vi "Output Powers.vi"(8 "error in":errorcluster, 9 "connection information":path, 10 "System Number":string, 11 "Arduino in":refnum<visa-resource-name>) -> (0 "error out":errorcluster, 3 "Arduino out":refnum<visa-resource-name>)   [LabVIEW 2024]
uses:
  <vilib>/addons/database/Connection.llb/DB Tools Open Connec (Path).vi
  <vilib>/addons/database/_DB Variant To Data/Database Variant To Data.xnode
  <instrlib>/Rohde&Schwarz Power Meter/Rohde&Schwarz Power Meter.lvlib
  <vilib>/addons/database/NI_Database_API.lvlib
panel:
  out "EFCVoltage":string
  out "OscVoltage":string
  out "Command Array":string[](array[string])
  out "OutputPower":string
  out "Temperature":string
  out "Nominal Frequency":string
  in  "DC_SN":string
  out "IsSine":bool=TRUE
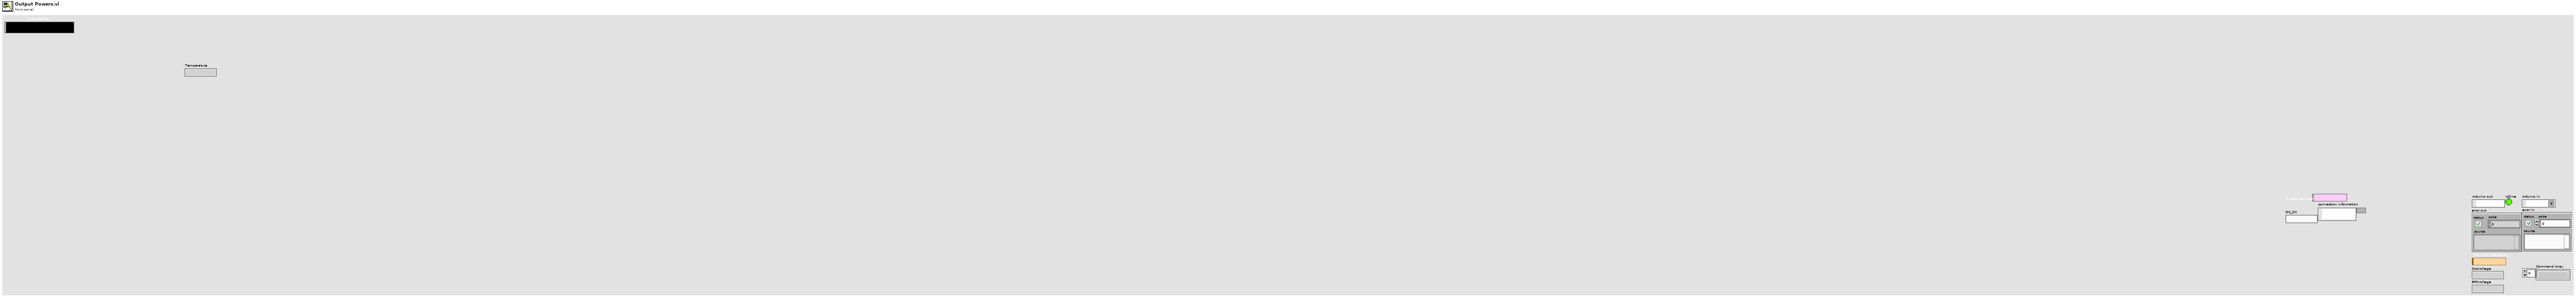
[diagram p1: front panel]
types:
  T1 = typedef "NI_Database_API.lvlib/Conn ObjectReference.ctl" = refnum<k1>
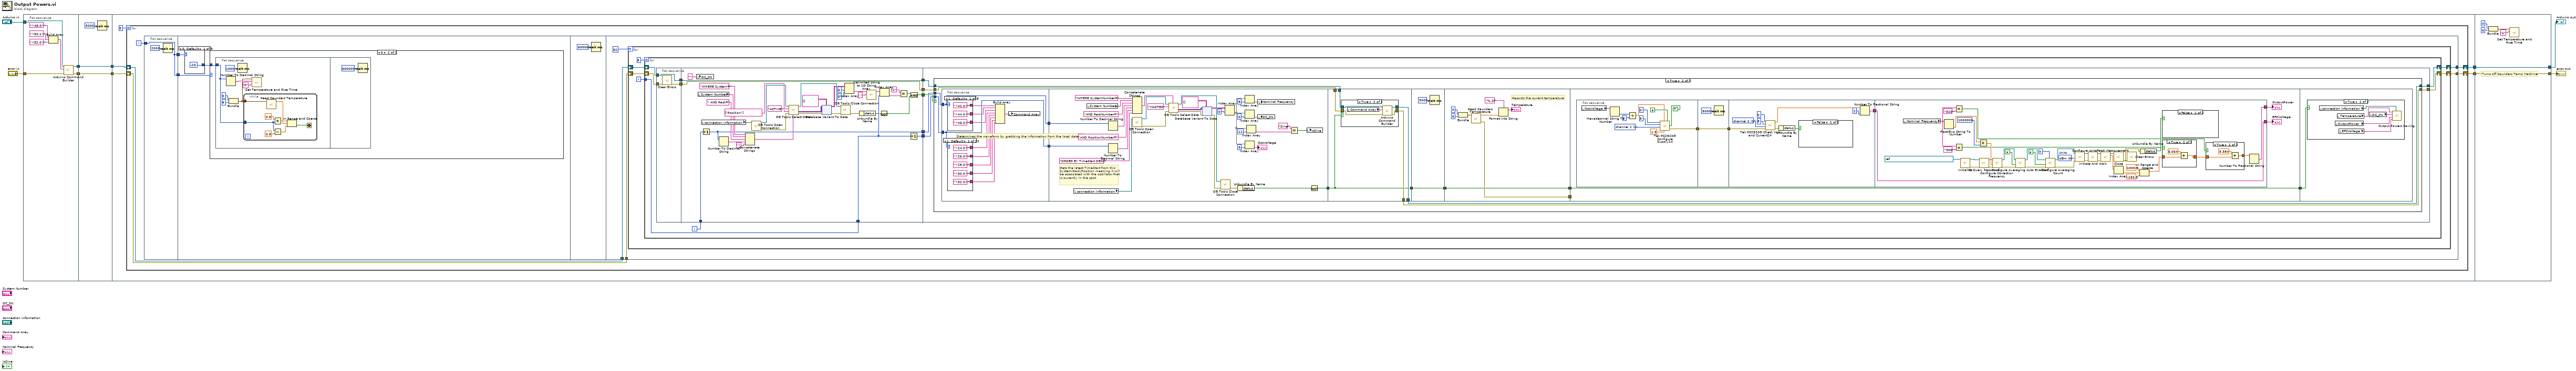
[diagram p0: block diagram]
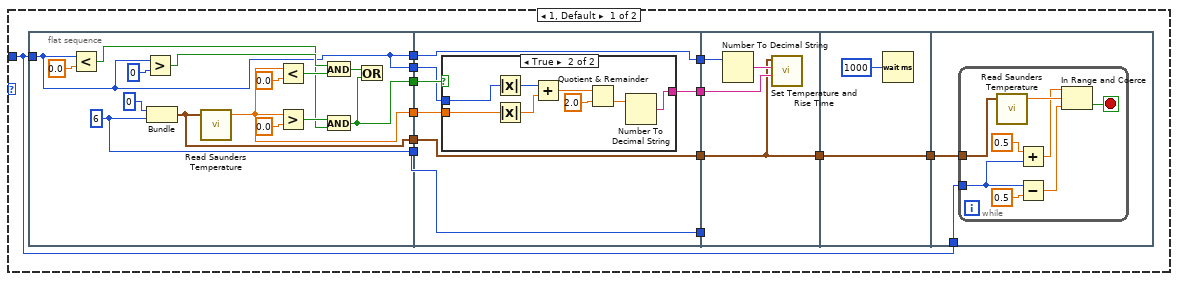
[diagram p2: hidden frame]
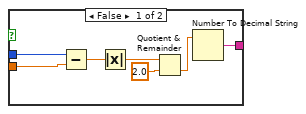
[diagram p3: hidden frame]
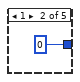
[diagram p4: hidden frame]
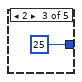
[diagram p5: hidden frame]
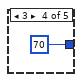
[diagram p6: hidden frame]
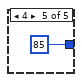
[diagram p7: hidden frame]
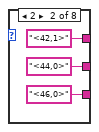
[diagram p9: hidden frame]
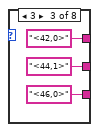
[diagram p10: hidden frame]
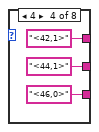
[diagram p11: hidden frame]
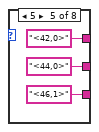
[diagram p12: hidden frame]
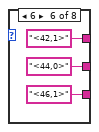
[diagram p13: hidden frame]
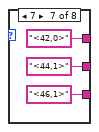
[diagram p14: hidden frame]
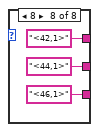
[diagram p15: hidden frame]
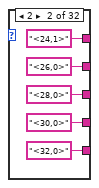
[diagram p16: hidden frame]
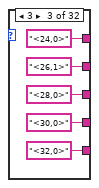
[diagram p17: hidden frame]
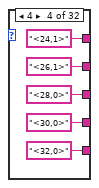
[diagram p18: hidden frame]
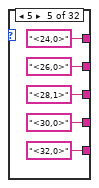
[diagram p19: hidden frame]
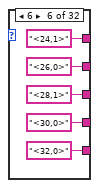
[diagram p20: hidden frame]
diagram:
  n1 = flat-sequence {
    tunnel: "Arduino in" -> [w18]
    tunnel: "error in" -> [w17]
    tunnel: [w15] -> w4
    tunnel: [w16] -> w2
    tunnel: w4 -> [w21]
    tunnel: [w21] -> w3
    tunnel: w2 -> [w20]
    tunnel: [w20] -> w1
    tunnel: [w22] -> w10
    tunnel: [w23] -> w9
    tunnel: w3 -> [w25]
    tunnel: w1 -> [w24]
    tunnel: [w638] -> w5
    tunnel: [w637] -> w6
    tunnel: w10 -> [w638]
    tunnel: w9 -> [w637]
    frame #0 {
      n2 = Build Array("<48,0>" ("string"), "<50,1>" ("string"), "<52,0>" ("string")) -> (w11:string[])
      n3 = call "Arduino Command Builder.vi"("error in"=w17, "Commands"=w11, "Arduino in"=w18) -> ("error out"=w15:errorcluster, "Arduino out"=w16:refnum<visa-resource-name>)  [unwired: 7 in]
    }
    frame #1 {
      n4 = Wait (ms)(milliseconds to wait=u32 5000) -> ()  [unwired: 1 out]
    }
    frame #2 {
      n5 = for {
        N: 5 -> [_]
        shift-right: [w30] -> w22
        shift-left: w25 -> [w33]
        shift-right: [w31] -> w23
        shift-left: w24 -> [w32]
        i -> [w29]
        n6 = flat-sequence {
          tunnel: w29 -> [w34]
          tunnel: [w34] -> w28
          tunnel: [w34] -> w27
          tunnel: w28 -> [w38]
          tunnel: w27 -> [w37]
          tunnel: w33 -> [w131]
          tunnel: w32 -> [w130]
          tunnel: [w129] -> w30
          tunnel: [w128] -> w31
          frame #0 {
            n7 = Wait (ms)(milliseconds to wait=u32 2000) -> ()  [unwired: 1 out]
          }
          frame #1 {
            n8 = case shown="0, Default" w38 {
              tunnel: [-20 0 25 70 85] -> w36
              frame 0, Default {
              }
              frame 1 {
              }
              frame 2 {
              }
              frame 3 {
              }
              frame 4 {
              }
            }
            n9 = case shown="0" w37 {
              tunnel: w36 -> [w39 w105]
              frame 1, Default {
                n10 = flat-sequence {
                  tunnel: w39 -> [w52]
                  tunnel: [w52] -> w51
                  tunnel: [w66] -> w50
                  tunnel: [w64] -> w49
                  tunnel: [w54] -> w48
                  tunnel: [w53] -> w47
                  tunnel: [w52] -> w46
                  tunnel: w51 -> [w73]
                  tunnel: [w73] -> w45
                  tunnel: [w67] -> w44
                  tunnel: w50 -> [w72]
                  tunnel: [w72] -> w43
                  tunnel: w49 -> [w71]
                  tunnel: [w71] -> w42
                  tunnel: w48 -> [w70]
                  tunnel: w47 -> [w69]
                  tunnel: w46 -> [w68]
                  tunnel: [w89] -> w41
                  tunnel: w45 -> [w91]
                  tunnel: w44 -> [w90]
                  tunnel: w43 -> [_]
                  tunnel: w42 -> [w89]
                  tunnel: [w93] -> w40
                  tunnel: w41 -> [w93]
                  tunnel: w39 -> [w96]
                  tunnel: w40 -> [w95]
                  frame #0 {
                    w66 = 6
                    n11 = Less?(x=w52, y=0.0) -> (x < y?=w58:bool)
                    n12 = Greater?(x=w52, y=0) -> (0:w61:bool)
                    n13 = Bundle(0, w66) -> (w64:cluster{i32, i32})  [unwired: 1 in]
                    n14 = call "Read Saunders Temperature.vi"("Device"=w64) -> ("Temperature"=w53:dbl)  [unwired: 3 in, 1 out]
                    n15 = Less?(x=w53, y=0.0) -> (x < y?=w60:bool)
                    n16 = Greater?(x=w53, y=0.0) -> (0:w59:bool)
                    n17 = And(x=w61, y=w60) -> (x .and. y?=w57:bool)
                    n18 = And(x=w59, y=w58) -> (x .and. y?=w54:bool)
                    n19 = Or(x=w57, y=w54) -> ()  [unwired: 1 out]
                  }
                  frame #1 {
                    n20 = case shown="True" w70 {
                      tunnel: w69 -> [w79 w87]
                      tunnel: w68 -> [w80 w88]
                      tunnel: [w75 w84] -> w67
                      frame False {
                        n21 = Subtract(x=w80, y=w79) -> (x-y=w78:dbl)
                        n22 = Absolute Value(x=w78) -> (abs(x)=w74:dbl)
                        n23 = Quotient & Remainder(x=w74, y=2.0) -> (floor(x/y)=w76:dbl)  [unwired: 1 out]
                        n24 = Number To Decimal String(number=w76) -> (decimal integer string=w75:string)  [unwired: 1 in]
                      }
                      frame True {
                        n25 = Absolute Value(x=w88) -> (abs(x)=w85:i32)
                        n26 = Absolute Value(x=w87) -> (abs(x)=w86:dbl)
                        n27 = Add(x=w85, y=w86) -> (x+y=w81:dbl)
                        n28 = Quotient & Remainder(x=w81, y=2.0) -> (floor(x/y)=w82:dbl)  [unwired: 1 out]
                        n29 = Number To Decimal String(number=w82) -> (decimal integer string=w84:string)  [unwired: 1 in]
                      }
                    }
                  }
                  frame #2 {
                    n30 = Number To Decimal String(number=w91) -> (decimal integer string=w92:string)  [unwired: 1 in]
                    n31 = call "Set Temperature and Rise Time.vi"("Slew Time String"=w90, "Temperature String"=w92, "Device"=w89) -> ()  [unwired: 3 in, 1 out]
                  }
                  frame #3 {
                    n32 = Wait (ms)(milliseconds to wait=u32 1000) -> ()  [unwired: 1 out]
                  }
                  frame #4 {
                    n33 = while {
                      tunnel: w95 -> [w104]
                      tunnel: w96 -> [w101]
                      stop <- w103 stop-if-true
                      n34 = call "Read Saunders Temperature.vi"("Device"=w104) -> ("Temperature"=w102:dbl)  [unwired: 3 in, 1 out]
                      n35 = Add(x=0.5, y=w101) -> (x+y=w97:dbl)
                      n36 = Subtract(x=w101, y=0.5) -> (x-y=w99:dbl)
                      n37 = In Range and Coerce(upper limit=w97, x=w102, lower limit=w99) -> (In Range?=w103:bool)  [unwired: 1 out]
                    }
                  }
                }
              }
              frame 0 {
                n38 = flat-sequence {
                  tunnel: w105 -> [w110]
                  frame #0 {
                    n39 = Number To Decimal String(number=w110) -> (decimal integer string=w112:string)  [unwired: 1 in]
                    n40 = Bundle(0, 6) -> (w106:cluster{i32, i32})  [unwired: 1 in]
                    n41 = Wait (ms)(milliseconds to wait=u32 1000) -> ()  [unwired: 1 out]
                    n42 = while {
                      tunnel: w106 -> [w120]
                      tunnel: w110 -> [w117]
                      stop <- w119 stop-if-true
                      n43 = call "Read Saunders Temperature.vi"("Device"=w120) -> ("Temperature"=w118:dbl)  [unwired: 3 in, 1 out]
                      n44 = Add(x=0.5, y=w117) -> (x+y=w113:dbl)
                      n45 = Subtract(x=w117, y=0.5) -> (x-y=w115:dbl)
                      n46 = In Range and Coerce(upper limit=w113, x=w118, lower limit=w115) -> (In Range?=w119:bool)  [unwired: 1 out]
                    }
                    n47 = call "Set Temperature and Rise Time.vi"("Slew Time String"="0", "Temperature String"=w112, "Device"=w106) -> ()  [unwired: 3 in, 1 out]
                  }
                  frame #1 {
                    n48 = Wait (ms)(milliseconds to wait=u32 600000) -> ()  [unwired: 1 out]
                  }
                }
              }
            }
          }
          frame #2 {
            n49 = Wait (ms)(milliseconds to wait=u32 60000) -> ()  [unwired: 1 out]
          }
          frame #3 {
            n50 = for {
              N: 32 -> [_]
              shift-right: [w134] -> w129
              shift-left: w131 -> [w137]
              shift-right: [w133] -> w128
              shift-left: w130 -> [w136]
              i -> [w135]
              n51 = for {
                N: 8 -> [_]
                shift-right: [w145] -> w134
                shift-left: w137 -> [w150]
                shift-right: [w141] -> w133
                shift-left: w136 -> [w149]
                tunnel: w135 -> [w148]
                i -> [w151]
                n52 = flat-sequence {
                  tunnel: w150 -> [w154]
                  tunnel: w149 -> [w153]
                  tunnel: [w153] -> w142
                  tunnel: [w152] -> w139
                  tunnel: w151 -> [w177]
                  tunnel: w148 -> [w176]
                  tunnel: [w175] -> w147
                  tunnel: [w174] -> w146
                  tunnel: [w173] -> w144
                  tunnel: [w172] -> w143
                  tunnel: w142 -> [w172]
                  tunnel: [w168] -> w140
                  tunnel: w139 -> [w173]
                  tunnel: [w240] -> w141
                  tunnel: [w239] -> w145
                  tunnel: w140 -> [w235]
                  tunnel: w143 -> [w236]
                  tunnel: w144 -> [w237]
                  tunnel: w146 -> [w238]
                  tunnel: w147 -> [w241]
                  frame #0 {
                    n53 = call <vilib>:"Clear Errors.vi"("error in (no error)"=w154) -> ("error out"=w152:errorcluster)  [unwired: 5 in, 1 out]
                  }
                  frame #1 {
                    n54 = local write "DC_SN"("" ("DC.SN")) -> ()
                    n55 = local read "System Number"() -> (w179:string)
                    n56 = local read "connection information"() -> (w157:path)
                    n57 = Increment(x=w177) -> (x+1=w175:i32)
                    n58 = Number To Decimal String(number=w175) -> (decimal integer string=w180:string)  [unwired: 1 in]
                    n59 = Concatenate Strings("WHERE System=" ("SQL Query"), w179, " AND Rack=", w180, ";" ("string")) -> (w156:string)
                    n60 = call-poly <vilib>:"DB Tools Open Connection.vi"("connection information"=w157) -> ("error out"=w166:errorcluster, "connection reference"=w167:T1)  [unwired: 7 in]
                    n61 = call <vilib>:"DB Tools Select Data.vi"("condition"=w156, "error in (no error)"=w166, "columns"=string[] ["Position"], "table"="ACTIVE", "connection reference"=w167) -> ("error out"=w163:errorcluster, "data"=w161:variant[][], "connection reference out"=w165:T1)  [unwired: 1 in]
                    n62 = xnode "Database Variant To Data"("database variant"=w161, "error in (no error)"=w163, "type"=string[][] [] ("DC.SN")) -> ("data"=w155:string[][], "error out"=w164:errorcluster)
                    n63 = call <vilib>:"DB Tools Close Connection.vi"("error in (no error)"=w164, "connection reference"=w165) -> ("error out"=w158:errorcluster)  [unwired: 5 in]
                    n64 = Index Array(array=w155, index (row)=0 ("disabled index (row)"), index (col)=0 ("disabled index (col)")) -> (element=w190:string)
                    n65 = Unbundle By Name(w158) -> ("status"=w171:bool)
                    n66 = call <vilib>:"Delimited String to 1D String Array.vi"("delimiter"=",", "delimited string"=w190) -> ("string array"=w187:string[])  [unwired: 9 in]
                    n67 = Not(x=w171) -> (.not. x?=w170:bool)
                    n68 = Index Array(array=w187, index=w176) -> (element=w186:string)
                    n69 = Equal?(x="1", y=w186) -> (x = y?=w169:bool)
                    n70 = Increment(x=w176) -> (x+1=w174:i32)
                    n71 = And(x=w169, y=w170) -> (x .and. y?=w168:bool)
                  }
                  frame #2 {
                    n72 = case shown="True" w235 {
                      tunnel: w241 -> [_ w257]
                      tunnel: w238 -> [_ w256]
                      tunnel: [w242 w253] -> w239
                      tunnel: w237 -> [w242 w255]
                      tunnel: w236 -> [w243 w254]
                      tunnel: [w243 w252] -> w240
                      frame False {
                      }
                      frame True {
                        n73 = flat-sequence {
                          tunnel: [w268] -> w245
                          tunnel: [w267] -> w244
                          tunnel: w257 -> [w268]
                          tunnel: w256 -> [w267]
                          tunnel: w245 -> [w480]
                          tunnel: w244 -> [w479]
                          tunnel: [w468] -> w251
                          tunnel: [w533] -> w253
                          tunnel: w255 -> [w535]
                          tunnel: w254 -> [w536]
                          tunnel: [w534] -> w252
                          tunnel: w251 -> [w532]
                          tunnel: [w532] -> w249
                          tunnel: [w544] -> w248
                          tunnel: w249 -> [w544]
                          tunnel: [w553] -> w247
                          tunnel: [w546] -> w246
                          tunnel: w248 -> [w546]
                          tunnel: [w559] -> w250
                          tunnel: w246 -> [w559]
                          tunnel: w247 -> [_]
                          tunnel: w250 -> [w631]
                          frame #0 {
                            # "Determines the waveform by grabbing the information from the local database"
                            n74 = case shown="1, Default" w268 {
                              tunnel: ["<42,0>" ("string") "<42,1>" ("string") "<42,0>" ("string") "<42,1>" ("string") "<42,0>" ("string") "<42,1>" ("string") "<42,0>" ("string") "<42,1>" ("string")] -> w260
                              tunnel: ["<44,0>" ("string") "<44,0>" ("string") "<44,1>" ("string") "<44,1>" ("string") "<44,0>" ("string") "<44,0>" ("string") "<44,1>" ("string") "<44,1>" ("string")] -> w259
                              tunnel: ["<46,0>" ("string") "<46,0>" ("string") "<46,0>" ("string") "<46,0>" ("string") "<46,1>" ("string") "<46,1>" ("string") "<46,1>" ("string") "<46,1>" ("string")] -> w258
                              frame 1, Default {
                              }
                              frame 2 {
                              }
                              frame 3 {
                              }
                              frame 4 {
                              }
                              frame 5 {
                              }
                              frame 6 {
                              }
                              frame 7 {
                              }
                              frame 8 {
                              }
                            }
                            n75 = case shown="1, Default" w267 {
                              tunnel: ["<32,0>" ("string") "<32,0>" ("string") "<32,0>" ("string") "<32,0>" ("string") "<32,0>" ("string") "<32,0>" ("string") "<32,0>" ("string") "<32,0>" ("string") "<32,0>" ("string") "<32,0>" ("string") "<32,0>" ("string") "<32,0>" ("string") "<32,0>" ("string") "<32,0>" ("string") "<32,0>" ("string") "<32,0>" ("string") "<32,1>" ("string") "<32,1>" ("string") "<32,1>" ("string") "<32,1>" ("string") "<32,1>" ("string") "<32,1>" ("string") "<32,1>" ("string") "<32,1>" ("string") "<32,1>" ("string") "<32,1>" ("string") "<32,1>" ("string") "<32,1>" ("string") "<32,1>" ("string") "<32,1>" ("string") "<32,1>" ("string") "<32,1>" ("string")] -> w262
                              tunnel: ["<30,0>" ("string") "<30,0>" ("string") "<30,0>" ("string") "<30,0>" ("string") "<30,0>" ("string") "<30,0>" ("string") "<30,0>" ("string") "<30,0>" ("string") "<30,1>" ("string") "<30,1>" ("string") "<30,1>" ("string") "<30,1>" ("string") "<30,1>" ("string") "<30,1>" ("string") "<30,1>" ("string") "<30,1>" ("string") "<30,0>" ("string") "<30,0>" ("string") "<30,0>" ("string") "<30,0>" ("string") "<30,0>" ("string") "<30,0>" ("string") "<30,0>" ("string") "<30,0>" ("string") "<30,1>" ("string") "<30,1>" ("string") "<30,1>" ("string") "<30,1>" ("string") "<30,1>" ("string") "<30,1>" ("string") "<30,1>" ("string") "<30,1>" ("string")] -> w263
                              tunnel: ["<28,0>" ("string") "<28,0>" ("string") "<28,0>" ("string") "<28,0>" ("string") "<28,1>" ("string") "<28,1>" ("string") "<28,1>" ("string") "<28,1>" ("string") "<28,0>" ("string") "<28,0>" ("string") "<28,0>" ("string") "<28,0>" ("string") "<28,1>" ("string") "<28,1>" ("string") "<28,1>" ("string") "<28,1>" ("string") "<28,0>" ("string") "<28,0>" ("string") "<28,0>" ("string") "<28,0>" ("string") "<28,1>" ("string") "<28,1>" ("string") "<28,1>" ("string") "<28,1>" ("string") "<28,0>" ("string") "<28,0>" ("string") "<28,0>" ("string") "<28,0>" ("string") "<28,1>" ("string") "<28,1>" ("string") "<28,1>" ("string") "<28,1>" ("string")] -> w264
                              tunnel: ["<26,0>" ("string") "<26,0>" ("string") "<26,1>" ("string") "<26,1>" ("string") "<26,0>" ("string") "<26,0>" ("string") "<26,1>" ("string") "<26,1>" ("string") "<26,0>" ("string") "<26,0>" ("string") "<26,1>" ("string") "<26,1>" ("string") "<26,0>" ("string") "<26,0>" ("string") "<26,1>" ("string") "<26,1>" ("string") "<26,0>" ("string") "<26,0>" ("string") "<26,1>" ("string") "<26,1>" ("string") "<26,0>" ("string") "<26,0>" ("string") "<26,1>" ("string") "<26,1>" ("string") "<26,0>" ("string") "<26,0>" ("string") "<26,1>" ("string") "<26,1>" ("string") "<26,0>" ("string") "<26,0>" ("string") "<26,1>" ("string") "<26,1>" ("string")] -> w265
                              tunnel: ["<24,0>" ("string") "<24,1>" ("string") "<24,0>" ("string") "<24,1>" ("string") "<24,0>" ("string") "<24,1>" ("string") "<24,0>" ("string") "<24,1>" ("string") "<24,0>" ("string") "<24,1>" ("string") "<24,0>" ("string") "<24,1>" ("string") "<24,0>" ("string") "<24,1>" ("string") "<24,0>" ("string") "<24,1>" ("string") "<24,0>" ("string") "<24,1>" ("string") "<24,0>" ("string") "<24,1>" ("string") "<24,0>" ("string") "<24,1>" ("string") "<24,0>" ("string") "<24,1>" ("string") "<24,0>" ("string") "<24,1>" ("string") "<24,0>" ("string") "<24,1>" ("string") "<24,0>" ("string") "<24,1>" ("string") "<24,0>" ("string") "<24,1>" ("string")] -> w266
                              frame 1, Default {
                              }
                              frame 2 {
                              }
                              frame 3 {
                              }
                              frame 4 {
                              }
                              frame 5 {
                              }
                              frame 6 {
                              }
                              frame 7 {
                              }
                              frame 8 {
                              }
                              frame 9 {
                              }
                              frame 10 {
                              }
                              frame 11 {
                              }
                              frame 12 {
                              }
                              frame 13 {
                              }
                              frame 14 {
                              }
                              frame 15 {
                              }
                              frame 16 {
                              }
                              frame 17 {
                              }
                              frame 18 {
                              }
                              frame 19 {
                              }
                              frame 20 {
                              }
                              frame 21 {
                              }
                              frame 22 {
                              }
                              frame 23 {
                              }
                              frame 24 {
                              }
                              frame 25 {
                              }
                              frame 26 {
                              }
                              frame 27 {
                              }
                              frame 28 {
                              }
                              frame 29 {
                              }
                              frame 30 {
                              }
                              frame 31 {
                              }
                              frame 32 {
                              }
                            }
                            n76 = Build Array(w260, w259, w258, w266, w265, w264, w263, w262) -> (w261:string[])
                            n77 = local write "Command Array"(w261) -> ()
                          }
                          frame #1 {
                            # "Gets the latest TimeStart from this System/Rack/Position meaning it will be associated with the oscillator that is currently in the spot"
                            n78 = local read "connection information"() -> (w456:path)
                            n79 = local read "System Number"() -> (w487:string)
                            n80 = Number To Decimal String(number=w480) -> (decimal integer string=w485:string)  [unwired: 1 in]
                            n81 = Number To Decimal String(number=w479) -> (decimal integer string=w486:string)  [unwired: 1 in]
                            n82 = Concatenate Strings("WHERE SystemNumber=" ("SQL Query"), w487, "AND RackNumber=" ("string"), w485, "AND PositionNumber=" ("string"), w486, "ORDER BY TimeStart DESC" ("string")) -> (w455:string)
                            n83 = call-poly <vilib>:"DB Tools Open Connection.vi"("connection information"=w456) -> ("error out"=w463:errorcluster, "connection reference"=w464:T1)  [unwired: 7 in]
                            n84 = call <vilib>:"DB Tools Select Data.vi"("condition"=w455, "error in (no error)"=w463, "table"="MASTER", "connection reference"=w464) -> ("error out"=w460:errorcluster, "data"=w458:variant[][], "connection reference out"=w462:T1)  [unwired: 2 in]
                            n85 = xnode "Database Variant To Data"("database variant"=w458, "error in (no error)"=w460, "type"=string[][] [] ("DC.SN")) -> ("data"=w454:string[][], "error out"=w461:errorcluster)
                            n86 = call <vilib>:"DB Tools Close Connection.vi"("error in (no error)"=w461, "connection reference"=w462) -> ("error out"=w453:errorcluster)  [unwired: 5 in]
                            n87 = Index Array(array=w454, index (row)=0 ("disabled index (row)")) -> (element=w466:string[])  [unwired: 1 in]
                            n88 = Unbundle By Name(w453) -> ("status"=w469:bool)
                            n89 = Index Array(array=w466, index=8) -> (element=w475:string)
                            n90 = Index Array(array=w466, index=0) -> (element=w474:string)
                            n91 = Index Array(array=w466, index=9) -> (element=→"OscVoltage":string)
                            n92 = Index Array(array=w466, index=11) -> (element=w476:string)
                            n93 = local write "Nominal Frequency"(w475) -> ()
                            n94 = local write "DC_SN"(w474) -> ()
                            n95 = Equal?(x="Sine", y=w476) -> (x = y?=w477:bool)
                            n96 = local write "IsSine"(w477) -> ()
                            n97 = Not(x=w469) -> (.not. x?=w468:bool)
                          }
                          frame #2 {
                            n98 = case shown="True" w532 {
                              tunnel: w536 -> [w538 w543]
                              tunnel: w535 -> [w537 w542]
                              tunnel: [w538 w541] -> w534
                              tunnel: [w537 w540] -> w533
                              frame False {
                              }
                              frame True {
                                n99 = local read "Command Array"() -> (w539:string[])
                                n100 = call "Arduino Command Builder.vi"("error in"=w542, "Commands"=w539, "Arduino in"=w543) -> ("error out"=w540:errorcluster, "Arduino out"=w541:refnum<visa-resource-name>)  [unwired: 7 in]
                              }
                            }
                          }
                          frame #3 {
                            n101 = Wait (ms)(milliseconds to wait=u32 3000 ("millisecond multiple")) -> ()  [unwired: 1 out]
                          }
                          frame #4 {
                            # "Records the current temperature"
                            n102 = Bundle(0, 6) -> (w552:cluster{i32, i32})  [unwired: 1 in]
                            n103 = call "Read Saunders Temperature.vi"("Device"=w552) -> ("error out 2"=w553:errorcluster, "Temperature"=w550:dbl)  [unwired: 3 in]
                            n104 = Format Into String(format string="%.2f" ("Format String"), w550) -> (resulting string=→"Temperature":string)  [unwired: 2 in, 1 out]
                          }
                          frame #5 {
                            n105 = flat-sequence {
                              tunnel: [w564] -> w557
                              tunnel: w557 -> [w572]
                              tunnel: [w572] -> w556
                              tunnel: w556 -> [w574]
                              tunnel: [w573] -> w554
                              tunnel: [w621] -> w558
                              tunnel: [w620] -> w555
                              tunnel: w554 -> [w620]
                              frame #0 {
                                w568 = u16 1 items=["channel 1", "channel 2", "channel 3"] ("channel (ch1:0)")
                                n106 = local read "OscVoltage"() -> (w562:string)
                                n107 = Hexadecimal String To Number(string=w562) -> (number=w561:u32)  [unwired: 2 in, 1 out]
                                n108 = Divide(x=w561, y=u32 2) -> (x/y=w563:dbl)
                                n109 = call "Tek PS2520G Configure Supply24.vi"("GPIB #"=u8 0, "voltage limit"=w563, "Address"=u8 8, "channel (ch1:0)"=w568, "current limit"=1.5, "Switch Output"=FALSE, "output (t:on)"=TRUE) -> ("error out"=w564:errorcluster)  [unwired: 1 in]
                              }
                              frame #1 {
                                n110 = Wait (ms)(milliseconds to wait=u32 5000) -> ()  [unwired: 1 out]
                              }
                              frame #2 {
                                w576 = u16 1 items=["channel 1", "channel 2", "channel 3"] ("channel (ch1:0)")
                                n111 = call "Tek PS2520G Check Volt and Current24.vi"("GPIB #"=u8 0, "Address"=u8 8, "channel (ch1:0)"=w576, "error in (no error)"=w574) -> ("actual output voltage"=w580:dbl, "error out"=w581:errorcluster)  [unwired: 2 in, 1 out]
                                n112 = Unbundle By Name(w581) -> ("status"=w579:bool)
                                n113 = case shown="False" w579 {
                                frame False {
                                }
                                frame True {
                                n114 = VISA Clear(VISA resource name=refnum<visa-resource-name> "GPIB0::8::INSTR") -> ()  [unwired: 1 in, 2 out]
                                }
                                }
                                n115 = Number To Fractional String(number=w580, precision (6)=i16 2) -> (F-format string=w573:string)  [unwired: 2 in]
                              }
                              frame #3 {
                                w594 = 0 items=["dBm", "W", "dBuv"]  # Units
                                n116 = local read "Nominal Frequency"() -> (w590:string)
                                n117 = Fract/Exp String To Number(string=w590) -> (number=w600:dbl)  [unwired: 3 in, 1 out]
                                n118 = Equal?(x=w590, y="320") -> (x = y?=w583:bool)
                                n119 = Equal?(x=w590, y="300") -> (x = y?=w584:bool)
                                n120 = call <instrlib>:"Initialize.vi"("VISA resource name"=refnum<visa-resource-name> "USB0::0x0AAD::0x00E2::113732::INSTR") -> ("VISA resource name out"=w605:refnum<visa-resource-name>, "error out"=w604:errorcluster)  [unwired: 13 in]
                                n121 = Multiply(x=w600, y=1000000) -> (x*y=w601:dbl)
                                n122 = call <instrlib>:"ID Query Response.vi"("error in (no error)"=w604, "VISA resource name"=w605) -> ("error out"=w602:errorcluster, "VISA resource name out"=w603:refnum<visa-resource-name>)  [unwired: 7 in, 1 out]
                                n123 = call <instrlib>:"Configure Correction Frequency.vi"("error in (no error)"=w602, "Correction Frequency (0Hz)"=w601, "VISA resource name"=w603) -> ("error out"=w611:errorcluster, "VISA resource name out"=w610:refnum<visa-resource-name>)  [unwired: 7 in]
                                n124 = call <instrlib>:"Configure Averaging Auto Enabled.vi"("error in (no error)"=w611, "Averaging Auto Enabled (Off)"=FALSE, "VISA resource name"=w610) -> ("error out"=w609:errorcluster, "VISA resource name out"=w608:refnum<visa-resource-name>)  [unwired: 7 in]
                                n125 = call <instrlib>:"Configure Averaging Count.vi"("Count (0)"=4, "error in (no error)"=w609, "Averaging State (Off)"=FALSE, "VISA resource name"=w608) -> ("error out"=w606:errorcluster, "VISA resource name out"=w607:refnum<visa-resource-name>)  [unwired: 6 in]
                                n126 = call <instrlib>:"Configure Units.vi"("error in (no error)"=w606, "Units (dBm)"=w594, "VISA resource name"=w607) -> ("error out"=w612:errorcluster, "VISA resource name out"=w613:refnum<visa-resource-name>)  [unwired: 7 in]
                                n127 = call <instrlib>:"Initiate And Wait.vi"("error in (no error)"=w612, "VISA resource name"=w613) -> ("error out"=w618:errorcluster, "VISA resource name out"=w616:refnum<visa-resource-name>)  [unwired: 8 in]
                                n128 = call <instrlib>:"Fetch Measurement.vi"("error in (no error)"=w618, "VISA resource name"=w616) -> ("Measurement"=w614:dbl[], "VISA resource name out"=w617:refnum<visa-resource-name>)  [unwired: 7 in, 1 out]
                                n129 = call <instrlib>:"Close.vi"("VISA resource name"=w617) -> ("error out"=w619:errorcluster)  [unwired: 10 in]
                                n130 = Index Array(array=w614) -> (element=w615:dbl)  [unwired: 1 in]
                                n131 = call <vilib>:"Clear Errors.vi"("error in (no error)"=w619) -> ()  [unwired: 5 in, 2 out]
                                n132 = In Range and Coerce(upper limit=1000.0, x=w615, lower limit=-150.0) -> (coerced(x)=w586:dbl)  [unwired: 1 out]
                                n133 = Unbundle By Name(w619) -> ("status"=w599:bool)
                                n134 = case shown="False" w599 {
                                frame False {
                                }
                                frame True {
                                n135 = VISA Clear(VISA resource name=refnum<visa-resource-name> "GPIB0::3::INSTR") -> ()  [unwired: 1 in, 2 out]
                                }
                                }
                                n136 = case shown="True" w584 {
                                tunnel: w586 -> [w626 w629]
                                tunnel: [w626 w628] -> w587
                                frame False {
                                }
                                frame True {
                                n137 = Add(x=6.064, y=w629) -> (x+y=w628:dbl)
                                }
                                }
                                n138 = case shown="True" w583 {
                                tunnel: w587 -> [w622 w624]
                                tunnel: [w622 w623] -> w585
                                frame False {
                                }
                                frame True {
                                n139 = Add(x=5.384, y=w624) -> (x+y=w623:dbl)
                                }
                                }
                                n140 = Number To Fractional String(number=w585) -> (F-format string=w621:string)  [unwired: 3 in]
                              }
                            }
                            "OutputPower" <- w558
                            "EFCVoltage" <- w555
                          }
                          frame #6 {
                            n141 = case shown="True" w631 {
                              frame False {
                              }
                              frame True {
                                n142 = local read "connection information"() -> (w632:path)
                                n143 = local read "OutputPower"() -> (w634:string)
                                n144 = local read "Temperature"() -> (w635:string)
                                n145 = local read "EFCVoltage"() -> (w633:string)
                                n146 = local read "DC_SN"() -> (w636:string)
                                n147 = call "Output Powers Saving.vi"("connection information"=w632, "EFCVoltage"=w633, "OutputPower"=w634, "DC_SN"=w636, "Temperature"=w635) -> ()  [unwired: 7 in]
                              }
                            }
                          }
                        }
                      }
                    }
                  }
                }
              }
            }
          }
        }
      }
    }
    frame #3 {
      # "Turns off Saunders Temp Machine"
      n148 = Bundle(0, 6) -> (w639:cluster{i32, i32})  [unwired: 1 in]
      n149 = call "Set Temperature and Rise Time.vi"("Temperature String"="o", "Device"=w639) -> ()  [unwired: 4 in, 1 out]
    }
  }
  "Arduino out" <- w6
  "error out" <- w5
